vi "Write Str to File.vi"(8 "error in":errorcluster, 10 "Str to Write":string, 11 "File Obs in":refnum<class "File Observer.lvclass">) -> (0 "error out":errorcluster, 3 "File Obs out":refnum<class "File Observer.lvclass">)   [LabVIEW 2015, in "File Observer.lvclass"]
uses:
  File Observer.lvclass
  File Observer.lvclass/File Observer.ctl
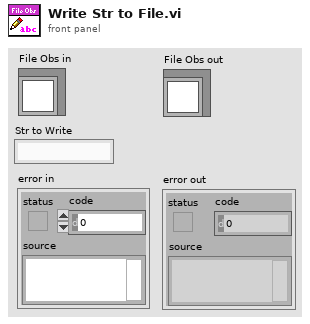
[diagram p1: front panel]
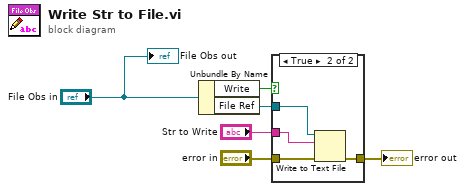
[diagram p0: block diagram]
diagram:
  n1 = Unbundle By Name("File Obs in") -> ("Write"=w1:bool, "File Ref"=w4:refnum<file>)
  n2 = case shown="True" w1 {
    tunnel: "Str to Write" -> [_ w11]
    tunnel: w4 -> [_ w10]
    tunnel: "error in" -> [w7 w9]
    tunnel: [w7 w8] -> w2
    frame False {
    }
    frame True {
      n3 = Write to Text File(file (use dialog)=w10, text=w11, error in=w9) -> (error out=w8:errorcluster)  [unwired: 1 in, 2 out]
    }
  }
  "error out" <- w2
  "File Obs out" <- "File Obs in"
